vi "Startup.vi"   [LabVIEW 2016]
uses:
  Manager.lvclass
  C:/Program Files (x86)/National Instruments/LabVIEW 2016/vi.lib/ActorFramework/Actor/Actor.lvclass
  <vilib>/ActorFramework/Actor/Actor.lvclass
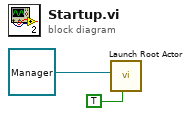
[diagram p0: block diagram]
diagram:
  n1 = call <vilib>:"Launch Root Actor.vi"("Open Actor Core front panel? (F)"=TRUE, "Actor"=refnum<class "Manager.lvclass"> refnum ("Manager.lvlib:Manager.lvclass")) -> ()  [unwired: 8 in, 2 out]
